vi "LSMcontroller_v58.vi"() -> ()   [LabVIEW 2015] (continued)
                    n4179 = call "2pparameters.vi"("command"="get") -> ("params out"=w943:T12)  [unwired: 1 in]
                    n4180 = Bundle By Name(cluster=w943, "Drawing Mode"=w916, "measpoints"=w932, "tt_cycles"=w934, "refreshbuffer"=w929, "refreshrate"=w928, "Vx-ref"=w935, "Vy-ref"=w937, "srate"=w926, "finite"=w939, "cont"=w938, "wavdet"=w940, "avpp"=w936, "srateAODO"=w933, "bufferAI"=w929, "bin"=w931, "Angle Img"=w923, "Vxminref"=w922, "Vxmaxref"=w921, "Vyminref"=w920, "Vymaxref"=w919, "Xpixels Img"=w918, "Ypixels Img"=w917, "Pel"=w915, "Vz-reset"=0.0, "AIoverride"=w913, "type"="Lifetime (contour)") -> (w941:T12)
                    n4181 = Reciprocal(x=w928) -> (1/x=w925:dbl)
                    n4182 = local write "refreshtime"(w925) -> ()
                    n4183 = call "2pparameters.vi"("Params in"=w941, "command"="set") -> ()  [unwired: 1 out]
                  }
                  frame "X-Y-Z-t movie" {
                  }
                  frame "linescan" {
                  }
                  frame "Timetrace" {
                    n4184 = local read "Vy-min draw"() -> (w953:dbl)
                    n4185 = local read "Vy-max draw"() -> (w952:dbl)
                    n4186 = local read "Vx-min draw"() -> (w955:dbl)
                    n4187 = local read "Vx-max draw"() -> (w954:dbl)
                    n4188 = local read "xpixels ref"() -> (w951:i32)
                    n4189 = local read "ypixels ref"() -> (w950:i32)
                    n4190 = local read "ROI Type"() -> (w949:u16)
                    n4191 = local read "srateAODOtt"() -> (w960:dbl)
                    n4192 = local read "# of frames"() -> (w965:i32)
                    n4193 = local read "refreshtime"() -> (w957:dbl)
                    n4194 = local read "Pel"() -> (w948:dbl)
                    n4195 = local read "bin"() -> (w963:dbl)
                    n4196 = local read "Override AI buffer"() -> (w946:bool)
                    n4197 = local read "finite samples"() -> (w972:bool)
                    n4198 = local read "srateAODOtt"() -> (w959:dbl)
                    n4199 = local read "srateAODOtt"() -> (w966:dbl)
                    n4200 = local read "continuous"() -> (w971:bool)
                    n4201 = local read "Angle ref"() -> (w956:dbl)
                    n4202 = local read "wavdet"() -> (w973:bool)
                    n4203 = local read "Vx-ref"() -> (w968:dbl)
                    n4204 = local read "Vy-ref"() -> (w970:dbl)
                    n4205 = local read "avpp"() -> (w969:i32)
                    n4206 = call "tt_timeandsamples.vi"("bin"=w963, "refreshtime"=w957, "srateAODOtt"=w960, "tot#ofsamples"=w965) -> ("refreshrate"=w961:dbl, "refreshbuffer"=w962:i32, "timetracecycles"=w967:i32)  [unwired: 5 in]
                    n4207 = local read "bin"() -> (w964:dbl)
                    n4208 = call "2pparameters.vi"("command"="get") -> ("params out"=w976:T12)  [unwired: 1 in]
                    n4209 = Bundle By Name(cluster=w976, "Drawing Mode"=w949, "measpoints"=w965, "tt_cycles"=w967, "refreshbuffer"=w962, "refreshrate"=w961, "Vx-ref"=w968, "Vy-ref"=w970, "srate"=w959, "finite"=w972, "cont"=w971, "wavdet"=w973, "avpp"=w969, "srateAODO"=w966, "bufferAI"=w962, "bin"=w964, "Angle Img"=w956, "Vxminref"=w955, "Vxmaxref"=w954, "Vyminref"=w953, "Vymaxref"=w952, "Xpixels Img"=w951, "Ypixels Img"=w950, "Pel"=w948, "Vz-reset"=0.0, "AIoverride"=w946, "type"="Timetrace") -> (w974:T12)
                    n4210 = Reciprocal(x=w961) -> (1/x=w958:dbl)
                    n4211 = local write "refreshtime"(w958) -> ()
                    n4212 = call "2pparameters.vi"("Params in"=w974, "command"="set") -> ()  [unwired: 1 out]
                  }
                  frame "Lifetime (point)" {
                  }
                }
              }
              frame #1 {
                w979 = FALSE ("wavdet")
                n4213 = call "2pparameters.vi"("command"="get") -> ("params out"=w983:T12)  [unwired: 1 in]
                n4214 = Bundle By Name(cluster=w983, "finite"=w979, "cont"=w979, "wavdet"=TRUE) -> (w980:T12)
                n4215 = call "2pparameters.vi"("Params in"=w980, "command"="set") -> ()  [unwired: 1 out]
              }
              frame #2 {
                n4216 = local read "DO channels"() -> (w988:u16)
                n4217 = call "2pparameters.vi"("command"="get") -> ("params out"=w990:T12)  [unwired: 1 in]
                n4218 = Unbundle By Name(w990) -> ("aDO"=w989:u32[])
                n4219 = Search 1D Array(1D array=w989, element=w988) -> (index of element=w986:i32)  [unwired: 1 in]
                n4220 = Greater?(x=w986, y=-1) -> (0:w985:bool)
                n4221 = case shown="True" w985 {
                  tunnel: w986 -> [_ w999]
                  frame False {
                  }
                  frame True {
                    n4222 = local read "Meastab"() -> (w993:enum32{"X-Y Image", "Linescan", "Timetrace"})
                    n4223 = local read "Digital padding value"() -> (w994:dbl)
                    n4224 = local read "Digital time offset (s)"() -> (w995:dbl)
                    n4225 = case shown="\"Timetrace\"" w993 {
                      tunnel: [w1000 w1001] -> w992
                      frame "X-Y Image", Default {
                        n4226 = local read "Sampling rate"() -> (w1000:dbl)
                      }
                      frame "Timetrace" {
                        n4227 = local read "srateAODOtt"() -> (w1001:dbl)
                      }
                    }
                    n4228 = local read "Digital Freq (Hz)"() -> (w997:dbl)
                    n4229 = local read "Digital phase (s)"() -> (w996:dbl)
                    n4230 = local read "Digital DC (%)"() -> (w998:dbl)
                    n4231 = call "replace DO wf param.vi"("Digital Freq (Hz)"=w997, "Digital DC (%)"=w998, "Digital phase"=w996, "Sampling frequency (Hz)"=w992, "Digital time offset (s)"=w995, "index of DO wave"=w999, "padding value"=w994) -> ()  [unwired: 4 in]
                  }
                }
              }
              frame #3 {
                n4232 = case shown="True" w1002 {
                  tunnel: w1003 -> [_ w1010]
                  frame False {
                  }
                  frame True {
                    n4233 = local read "Meastab"() -> (w1007:enum32{"X-Y Image", "Linescan", "Timetrace"})
                    n4234 = call "waveformparamsv2.vi"("command"="get") -> ("Params out"=w1026:T16)  [unwired: 4 in, 2 out]
                    n4235 = Unbundle By Name(w1026) -> ("DO parameters"=w1025:T19)
                    n4236 = property on="refwf" class="Ring (strict)"() -> ("RingText.Text"=w1032:string)  [unwired: 2 in, 2 out]
                    n4237 = case shown="\"Timetrace\"" w1007 {
                      tunnel: [w1033 w1034] -> w1006
                      frame "X-Y Image", Default {
                        n4238 = local read "Sampling rate"() -> (w1033:dbl)
                      }
                      frame "Timetrace" {
                        n4239 = local read "srateAODOtt"() -> (w1034:dbl)
                      }
                    }
                    n4240 = call "waveformsAObuffer.vi"("command"="get") -> ("AO wf out"=w1030:waveform(dbl)[])  [unwired: 1 in]
                    n4241 = call "waveformsDObuffer.vi"("command"="get") -> ("DO wf out"=w1028:digitalwaveform[])  [unwired: 1 in]
                    n4242 = call "referfencesize.vi"("Digital waveforms in"=w1028, "Analog waveforms in"=w1030, "reference waveforms to"=w1032) -> ("number of samples"=w1023:i32)  [unwired: 2 in]
                    n4243 = Index Array(array=w1025, index=w1010) -> (element=w1024:T20)
                    n4244 = call "waveformsDObuffer.vi"("command"="get") -> ("DO wf out"=w1020:digitalwaveform[])  [unwired: 1 in]
                    n4245 = call "simple digital from wf params.vi"("waveform params"=w1024, "number of samples"=w1023) -> ("digital waveform"=w1022:digitalwaveform)
                    n4246 = property on="refwf" class="Ring (strict)"() -> ("RingText.Text"=w1012:string)  [unwired: 2 in, 2 out]
                    n4247 = Replace Array Subset(array=w1020, new element=w1022, index=w1010) -> (w1011:digitalwaveform[])
                    n4248 = call "waveformsAObuffer.vi"("command"="get") -> ("AO wf out"=w1019:waveform(dbl)[])  [unwired: 1 in]
                    n4249 = local read "wavdet"() -> (w1009:bool)
                    n4250 = call "correctwaveformsizetemp.vi"("new sampling frequency (Hz)"=w1006, "start"=FALSE, "reference waveforms to"=w1012, "Analog waveforms in"=w1019, "stop"=FALSE, "Digital waveforms in"=w1011) -> ("analog wf out"=w1015:waveform(dbl)[], "Digital wf out"=w1013:digitalwaveform[], "measpoints"=w1008:i32)
                    n4251 = local write "Analog Lines Plot"(w1015) -> ()
                    n4252 = call "GetNumCamFramesv2.vi"("Digital Waveform Graph"=w1013) -> ("Numeric"=w1014:i32)  [unwired: 10 in]
                    n4253 = local write "Digital Lines Plot"(w1013) -> ()
                    n4254 = case shown="True" w1009 {
                      tunnel: w1008 -> [_ w1035]
                      frame False {
                      }
                      frame True {
                        n4255 = local write "# of frames"(w1035) -> ()
                      }
                    }
                    n4256 = call "waveformsAObuffer.vi"("AO wf in"=w1015, "command"="set") -> ()  [unwired: 1 out]
                    n4257 = call "waveformsDObuffer.vi"("DO wf in"=w1013, "command"="set") -> ()  [unwired: 1 out]
                    n4258 = local write "Total Camera Frames"(w1014) -> ()
                  }
                }
              }
              frame #4 {
                n4259 = local read "finite samples"() -> (w1036:bool)
                n4260 = local read "continuous"() -> (w1037:bool)
                n4261 = local read "wavdet"() -> (w1038:bool)
                n4262 = call "2pparameters.vi"("command"="get") -> ("params out"=w1041:T12)  [unwired: 1 in]
                n4263 = Bundle By Name(cluster=w1041, "finite"=w1036, "cont"=w1037, "wavdet"=w1038) -> (w1039:T12)
                n4264 = call "2pparameters.vi"("Params in"=w1039, "command"="set") -> ()  [unwired: 1 out]
              }
            }
          }
          event "refwf": Value Change {
            n4265 = event-data() -> ()  [unwired: 1 in, 6 out]
            n4266 = stacked-sequence {
              frame #0 {
                n4267 = local read "Measurement"() -> (w1043:T5)
                n4268 = case shown="\"X-Y-t movie\", Default" w1043 {
                  frame "X-Y-t movie", Default {
                    n4269 = local read "avpp"() -> (w1064:i32)
                    n4270 = local read "Angle ref"() -> (w1063:dbl)
                    n4271 = local read "ROI Type"() -> (w1062:u16)
                    n4272 = local read "xpixels ref"() -> (w1059:i32)
                    n4273 = local read "Vx-min ref"() -> (w1058:dbl)
                    n4274 = local read "Vx-max ref"() -> (w1057:dbl)
                    n4275 = local read "ypixels ref"() -> (w1055:i32)
                    n4276 = local read "Vy-min ref"() -> (w1056:dbl)
                    n4277 = local read "Vy-max ref"() -> (w1052:dbl)
                    n4278 = local read "Sampling rate"() -> (w1046:dbl)
                    n4279 = local read "finite samples"() -> (w1047:bool)
                    n4280 = local read "continuous"() -> (w1050:bool)
                    n4281 = local read "wavdet"() -> (w1051:bool)
                    n4282 = local read "# of frames"() -> (w1049:i32)
                    n4283 = local read "maxbufferAI"() -> (w1048:i32)
                    n4284 = local read "Override AI buffer"() -> (w1044:bool)
                    n4285 = call "2pparameters.vi"("command"="get") -> ("params out"=w1061:T12)  [unwired: 1 in]
                    n4286 = Bundle By Name(cluster=w1061, "type"="X-Y-t movie", "avpp"=w1064, "Angle Img"=w1063, "Xpixels Img"=w1059, "Vx-min Img"=w1058, "VX-max Img"=w1057, "Ypixels Img"=w1055, "Vy-min Img"=w1056, "Vy-max Img"=w1052, "srate"=w1046, "srate Img"=w1046, "finite"=w1047, "cont"=w1050, "wavdet"=w1051, "measpoints"=w1049, "maxbufferAI"=w1048, "Drawing Mode"=w1062, "Vz-reset"=0.0, "AIoverride"=w1044) -> (w1053:T12)
                    n4287 = call "2pparameters.vi"("Params in"=w1053, "command"="set") -> ()  [unwired: 1 out]
                  }
                  frame "X-Y-Z stack" {
                    n4288 = call "2pparameters.vi"("command"="get") -> ("params out"=w1068:T12)  [unwired: 1 in]
                    n4289 = Bundle By Name(cluster=w1068, "type"="X-Y-Z stack") -> (w1066:T12)
                    n4290 = call "2pparameters.vi"("Params in"=w1066, "command"="set") -> ()  [unwired: 1 out]
                  }
                  frame "Lifetime (scan)" {
                    n4291 = call "2pparameters.vi"("command"="get") -> ("params out"=w1073:T12)  [unwired: 1 in]
                    n4292 = Bundle By Name(cluster=w1073, "type"="Lifetime (scan)") -> (w1071:T12)
                    n4293 = call "2pparameters.vi"("Params in"=w1071, "command"="set") -> ()  [unwired: 1 out]
                  }
                  frame "Lifetime (contour)" {
                    n4294 = local read "Vy-min draw"() -> (w1083:dbl)
                    n4295 = local read "Vy-max draw"() -> (w1082:dbl)
                    n4296 = local read "Vx-min draw"() -> (w1085:dbl)
                    n4297 = local read "Vx-max draw"() -> (w1084:dbl)
                    n4298 = local read "xpixels ref"() -> (w1081:i32)
                    n4299 = local read "ypixels ref"() -> (w1080:i32)
                    n4300 = local read "ROI Type"() -> (w1079:u16)
                    n4301 = local read "srateAODOtt"() -> (w1090:dbl)
                    n4302 = local read "# of frames"() -> (w1095:i32)
                    n4303 = local read "refreshtime"() -> (w1087:dbl)
                    n4304 = local read "Pel"() -> (w1078:dbl)
                    n4305 = local read "bin"() -> (w1093:dbl)
                    n4306 = local read "Override AI buffer"() -> (w1076:bool)
                    n4307 = local read "finite samples"() -> (w1102:bool)
                    n4308 = local read "srateAODOtt"() -> (w1089:dbl)
                    n4309 = local read "srateAODOtt"() -> (w1096:dbl)
                    n4310 = local read "continuous"() -> (w1101:bool)
                    n4311 = local read "Angle ref"() -> (w1086:dbl)
                    n4312 = local read "wavdet"() -> (w1103:bool)
                    n4313 = local read "Vx-ref"() -> (w1098:dbl)
                    n4314 = local read "Vy-ref"() -> (w1100:dbl)
                    n4315 = local read "avpp"() -> (w1099:i32)
                    n4316 = call "tt_timeandsamples.vi"("bin"=w1093, "refreshtime"=w1087, "srateAODOtt"=w1090, "tot#ofsamples"=w1095) -> ("refreshrate"=w1091:dbl, "refreshbuffer"=w1092:i32, "timetracecycles"=w1097:i32)  [unwired: 5 in]
                    n4317 = local read "bin"() -> (w1094:dbl)
                    n4318 = call "2pparameters.vi"("command"="get") -> ("params out"=w1106:T12)  [unwired: 1 in]
                    n4319 = Bundle By Name(cluster=w1106, "Drawing Mode"=w1079, "measpoints"=w1095, "tt_cycles"=w1097, "refreshbuffer"=w1092, "refreshrate"=w1091, "Vx-ref"=w1098, "Vy-ref"=w1100, "srate"=w1089, "finite"=w1102, "cont"=w1101, "wavdet"=w1103, "avpp"=w1099, "srateAODO"=w1096, "bufferAI"=w1092, "bin"=w1094, "Angle Img"=w1086, "Vxminref"=w1085, "Vxmaxref"=w1084, "Vyminref"=w1083, "Vymaxref"=w1082, "Xpixels Img"=w1081, "Ypixels Img"=w1080, "Pel"=w1078, "Vz-reset"=0.0, "AIoverride"=w1076, "type"="Lifetime (contour)") -> (w1104:T12)
                    n4320 = Reciprocal(x=w1091) -> (1/x=w1088:dbl)
                    n4321 = local write "refreshtime"(w1088) -> ()
                    n4322 = call "2pparameters.vi"("Params in"=w1104, "command"="set") -> ()  [unwired: 1 out]
                  }
                  frame "X-Y-Z-t movie" {
                  }
                  frame "linescan" {
                  }
                  frame "Timetrace" {
                    n4323 = local read "Vy-min draw"() -> (w1116:dbl)
                    n4324 = local read "Vy-max draw"() -> (w1115:dbl)
                    n4325 = local read "Vx-min draw"() -> (w1118:dbl)
                    n4326 = local read "Vx-max draw"() -> (w1117:dbl)
                    n4327 = local read "xpixels ref"() -> (w1114:i32)
                    n4328 = local read "ypixels ref"() -> (w1113:i32)
                    n4329 = local read "ROI Type"() -> (w1112:u16)
                    n4330 = local read "srateAODOtt"() -> (w1123:dbl)
                    n4331 = local read "# of frames"() -> (w1128:i32)
                    n4332 = local read "refreshtime"() -> (w1120:dbl)
                    n4333 = local read "Pel"() -> (w1111:dbl)
                    n4334 = local read "bin"() -> (w1126:dbl)
                    n4335 = local read "Override AI buffer"() -> (w1109:bool)
                    n4336 = local read "finite samples"() -> (w1135:bool)
                    n4337 = local read "srateAODOtt"() -> (w1122:dbl)
                    n4338 = local read "srateAODOtt"() -> (w1129:dbl)
                    n4339 = local read "continuous"() -> (w1134:bool)
                    n4340 = local read "Angle ref"() -> (w1119:dbl)
                    n4341 = local read "wavdet"() -> (w1136:bool)
                    n4342 = local read "Vx-ref"() -> (w1131:dbl)
                    n4343 = local read "Vy-ref"() -> (w1133:dbl)
                    n4344 = local read "avpp"() -> (w1132:i32)
                    n4345 = call "tt_timeandsamples.vi"("bin"=w1126, "refreshtime"=w1120, "srateAODOtt"=w1123, "tot#ofsamples"=w1128) -> ("refreshrate"=w1124:dbl, "refreshbuffer"=w1125:i32, "timetracecycles"=w1130:i32)  [unwired: 5 in]
                    n4346 = local read "bin"() -> (w1127:dbl)
                    n4347 = call "2pparameters.vi"("command"="get") -> ("params out"=w1139:T12)  [unwired: 1 in]
                    n4348 = Bundle By Name(cluster=w1139, "Drawing Mode"=w1112, "measpoints"=w1128, "tt_cycles"=w1130, "refreshbuffer"=w1125, "refreshrate"=w1124, "Vx-ref"=w1131, "Vy-ref"=w1133, "srate"=w1122, "finite"=w1135, "cont"=w1134, "wavdet"=w1136, "avpp"=w1132, "srateAODO"=w1129, "bufferAI"=w1125, "bin"=w1127, "Angle Img"=w1119, "Vxminref"=w1118, "Vxmaxref"=w1117, "Vyminref"=w1116, "Vymaxref"=w1115, "Xpixels Img"=w1114, "Ypixels Img"=w1113, "Pel"=w1111, "Vz-reset"=0.0, "AIoverride"=w1109, "type"="Timetrace") -> (w1137:T12)
                    n4349 = Reciprocal(x=w1124) -> (1/x=w1121:dbl)
                    n4350 = local write "refreshtime"(w1121) -> ()
                    n4351 = call "2pparameters.vi"("Params in"=w1137, "command"="set") -> ()  [unwired: 1 out]
                  }
                  frame "Lifetime (point)" {
                  }
                }
              }
              frame #1 {
                w1142 = FALSE ("wavdet")
                n4352 = call "2pparameters.vi"("command"="get") -> ("params out"=w1146:T12)  [unwired: 1 in]
                n4353 = Bundle By Name(cluster=w1146, "finite"=w1142, "cont"=w1142, "wavdet"=TRUE) -> (w1143:T12)
                n4354 = call "2pparameters.vi"("Params in"=w1143, "command"="set") -> ()  [unwired: 1 out]
              }
              frame #2 {
                n4355 = local read "Meastab"() -> (w1151:enum32{"X-Y Image", "Linescan", "Timetrace"})
                n4356 = property on="refwf" class="Ring (strict)"() -> ("RingText.Text"=w1154:string)  [unwired: 2 in, 2 out]
                n4357 = case shown="\"Timetrace\"" w1151 {
                  tunnel: [w1164 w1165] -> w1150
                  frame "X-Y Image", Default {
                    n4358 = local read "Sampling rate"() -> (w1164:dbl)
                  }
                  frame "Timetrace" {
                    n4359 = local read "srateAODOtt"() -> (w1165:dbl)
                  }
                }
                n4360 = call "waveformsAObuffer.vi"("command"="get") -> ("AO wf out"=w1163:waveform(dbl)[])  [unwired: 1 in]
                n4361 = local read "wavdet"() -> (w1153:bool)
                n4362 = call "waveformsDObuffer.vi"("command"="get") -> ("DO wf out"=w1159:digitalwaveform[])  [unwired: 1 in]
                n4363 = call "correctwaveformsizetemp.vi"("new sampling frequency (Hz)"=w1150, "start"=FALSE, "reference waveforms to"=w1154, "Analog waveforms in"=w1163, "stop"=FALSE, "Digital waveforms in"=w1159) -> ("analog wf out"=w1157:waveform(dbl)[], "Digital wf out"=w1155:digitalwaveform[], "measpoints"=w1152:i32)
                n4364 = local write "Analog Lines Plot"(w1157) -> ()
                n4365 = call "GetNumCamFramesv2.vi"("Digital Waveform Graph"=w1155) -> ("Numeric"=w1156:i32)  [unwired: 10 in]
                n4366 = local write "Digital Lines Plot"(w1155) -> ()
                n4367 = call "waveformsDObuffer.vi"("DO wf in"=w1155, "command"="set") -> ()  [unwired: 1 out]
                n4368 = call "waveformsAObuffer.vi"("AO wf in"=w1157, "command"="set") -> ()  [unwired: 1 out]
                n4369 = local write "Total Camera Frames"(w1156) -> ()
                n4370 = case shown="True" w1153 {
                  tunnel: w1152 -> [_ w1166]
                  frame False {
                  }
                  frame True {
                    n4371 = local write "# of frames"(w1166) -> ()
                  }
                }
              }
              frame #3 {
                n4372 = local read "finite samples"() -> (w1167:bool)
                n4373 = local read "continuous"() -> (w1168:bool)
                n4374 = local read "wavdet"() -> (w1169:bool)
                n4375 = call "2pparameters.vi"("command"="get") -> ("params out"=w1172:T12)  [unwired: 1 in]
                n4376 = Bundle By Name(cluster=w1172, "finite"=w1167, "cont"=w1168, "wavdet"=w1169) -> (w1170:T12)
                n4377 = call "2pparameters.vi"("Params in"=w1170, "command"="set") -> ()  [unwired: 1 out]
              }
            }
          }
          event "Start amplitude (V)", "Cycles", "Baseline (V)", "Step size (V)", "DC (%)", "Period (ms)", "Repeats", "Pulses", "phase shift (ms)": Value Change {
            n4378 = event-data() -> ()  [unwired: 1 in, 6 out]
            n4379 = stacked-sequence {
              seq-local: [_ _ w1280 _ _] -> [_ _ _ w1302 _]
              seq-local: [_ _ w1279 _ _] -> [_ _ _ w1301 _]
              frame #0 {
                n4380 = local read "Measurement"() -> (w1174:T5)
                n4381 = case shown="\"X-Y-t movie\", Default" w1174 {
                  frame "X-Y-t movie", Default {
                    n4382 = local read "avpp"() -> (w1195:i32)
                    n4383 = local read "Angle ref"() -> (w1194:dbl)
                    n4384 = local read "ROI Type"() -> (w1193:u16)
                    n4385 = local read "xpixels ref"() -> (w1190:i32)
                    n4386 = local read "Vx-min ref"() -> (w1189:dbl)
                    n4387 = local read "Vx-max ref"() -> (w1188:dbl)
                    n4388 = local read "ypixels ref"() -> (w1186:i32)
                    n4389 = local read "Vy-min ref"() -> (w1187:dbl)
                    n4390 = local read "Vy-max ref"() -> (w1183:dbl)
                    n4391 = local read "Sampling rate"() -> (w1177:dbl)
                    n4392 = local read "finite samples"() -> (w1178:bool)
                    n4393 = local read "continuous"() -> (w1181:bool)
                    n4394 = local read "wavdet"() -> (w1182:bool)
                    n4395 = local read "# of frames"() -> (w1180:i32)
                    n4396 = local read "maxbufferAI"() -> (w1179:i32)
                    n4397 = local read "Override AI buffer"() -> (w1175:bool)
                    n4398 = call "2pparameters.vi"("command"="get") -> ("params out"=w1192:T12)  [unwired: 1 in]
                    n4399 = Bundle By Name(cluster=w1192, "type"="X-Y-t movie", "avpp"=w1195, "Angle Img"=w1194, "Xpixels Img"=w1190, "Vx-min Img"=w1189, "VX-max Img"=w1188, "Ypixels Img"=w1186, "Vy-min Img"=w1187, "Vy-max Img"=w1183, "srate"=w1177, "srate Img"=w1177, "finite"=w1178, "cont"=w1181, "wavdet"=w1182, "measpoints"=w1180, "maxbufferAI"=w1179, "Drawing Mode"=w1193, "Vz-reset"=0.0, "AIoverride"=w1175) -> (w1184:T12)
                    n4400 = call "2pparameters.vi"("Params in"=w1184, "command"="set") -> ()  [unwired: 1 out]
                  }
                  frame "X-Y-Z stack" {
                    n4401 = call "2pparameters.vi"("command"="get") -> ("params out"=w1199:T12)  [unwired: 1 in]
                    n4402 = Bundle By Name(cluster=w1199, "type"="X-Y-Z stack") -> (w1197:T12)
                    n4403 = call "2pparameters.vi"("Params in"=w1197, "command"="set") -> ()  [unwired: 1 out]
                  }
                  frame "Lifetime (scan)" {
                    n4404 = call "2pparameters.vi"("command"="get") -> ("params out"=w1204:T12)  [unwired: 1 in]
                    n4405 = Bundle By Name(cluster=w1204, "type"="Lifetime (scan)") -> (w1202:T12)
                    n4406 = call "2pparameters.vi"("Params in"=w1202, "command"="set") -> ()  [unwired: 1 out]
                  }
                  frame "Lifetime (contour)" {
                    n4407 = local read "Vy-min draw"() -> (w1214:dbl)
                    n4408 = local read "Vy-max draw"() -> (w1213:dbl)
                    n4409 = local read "Vx-min draw"() -> (w1216:dbl)
                    n4410 = local read "Vx-max draw"() -> (w1215:dbl)
                    n4411 = local read "xpixels ref"() -> (w1212:i32)
                    n4412 = local read "ypixels ref"() -> (w1211:i32)
                    n4413 = local read "ROI Type"() -> (w1210:u16)
                    n4414 = local read "srateAODOtt"() -> (w1221:dbl)
                    n4415 = local read "# of frames"() -> (w1226:i32)
                    n4416 = local read "refreshtime"() -> (w1218:dbl)
                    n4417 = local read "Pel"() -> (w1209:dbl)
                    n4418 = local read "bin"() -> (w1224:dbl)
                    n4419 = local read "Override AI buffer"() -> (w1207:bool)
                    n4420 = local read "finite samples"() -> (w1233:bool)
                    n4421 = local read "srateAODOtt"() -> (w1220:dbl)
                    n4422 = local read "srateAODOtt"() -> (w1227:dbl)
                    n4423 = local read "continuous"() -> (w1232:bool)
                    n4424 = local read "Angle ref"() -> (w1217:dbl)
                    n4425 = local read "wavdet"() -> (w1234:bool)
                    n4426 = local read "Vx-ref"() -> (w1229:dbl)
                    n4427 = local read "Vy-ref"() -> (w1231:dbl)
                    n4428 = local read "avpp"() -> (w1230:i32)
                    n4429 = call "tt_timeandsamples.vi"("bin"=w1224, "refreshtime"=w1218, "srateAODOtt"=w1221, "tot#ofsamples"=w1226) -> ("refreshrate"=w1222:dbl, "refreshbuffer"=w1223:i32, "timetracecycles"=w1228:i32)  [unwired: 5 in]
                    n4430 = local read "bin"() -> (w1225:dbl)
                    n4431 = call "2pparameters.vi"("command"="get") -> ("params out"=w1237:T12)  [unwired: 1 in]
                    n4432 = Bundle By Name(cluster=w1237, "Drawing Mode"=w1210, "measpoints"=w1226, "tt_cycles"=w1228, "refreshbuffer"=w1223, "refreshrate"=w1222, "Vx-ref"=w1229, "Vy-ref"=w1231, "srate"=w1220, "finite"=w1233, "cont"=w1232, "wavdet"=w1234, "avpp"=w1230, "srateAODO"=w1227, "bufferAI"=w1223, "bin"=w1225, "Angle Img"=w1217, "Vxminref"=w1216, "Vxmaxref"=w1215, "Vyminref"=w1214, "Vymaxref"=w1213, "Xpixels Img"=w1212, "Ypixels Img"=w1211, "Pel"=w1209, "Vz-reset"=0.0, "AIoverride"=w1207, "type"="Lifetime (contour)") -> (w1235:T12)
                    n4433 = Reciprocal(x=w1222) -> (1/x=w1219:dbl)
                    n4434 = local write "refreshtime"(w1219) -> ()
                    n4435 = call "2pparameters.vi"("Params in"=w1235, "command"="set") -> ()  [unwired: 1 out]
                  }
                  frame "X-Y-Z-t movie" {
                  }
                  frame "linescan" {
                  }
                  frame "Timetrace" {
                    n4436 = local read "Vy-min draw"() -> (w1247:dbl)
                    n4437 = local read "Vy-max draw"() -> (w1246:dbl)
                    n4438 = local read "Vx-min draw"() -> (w1249:dbl)
                    n4439 = local read "Vx-max draw"() -> (w1248:dbl)
                    n4440 = local read "xpixels ref"() -> (w1245:i32)
                    n4441 = local read "ypixels ref"() -> (w1244:i32)
                    n4442 = local read "ROI Type"() -> (w1243:u16)
                    n4443 = local read "srateAODOtt"() -> (w1254:dbl)
                    n4444 = local read "# of frames"() -> (w1259:i32)
                    n4445 = local read "refreshtime"() -> (w1251:dbl)
                    n4446 = local read "Pel"() -> (w1242:dbl)
                    n4447 = local read "bin"() -> (w1257:dbl)
                    n4448 = local read "Override AI buffer"() -> (w1240:bool)
                    n4449 = local read "finite samples"() -> (w1266:bool)
                    n4450 = local read "srateAODOtt"() -> (w1253:dbl)
                    n4451 = local read "srateAODOtt"() -> (w1260:dbl)
                    n4452 = local read "continuous"() -> (w1265:bool)
                    n4453 = local read "Angle ref"() -> (w1250:dbl)
                    n4454 = local read "wavdet"() -> (w1267:bool)
                    n4455 = local read "Vx-ref"() -> (w1262:dbl)
                    n4456 = local read "Vy-ref"() -> (w1264:dbl)
                    n4457 = local read "avpp"() -> (w1263:i32)
                    n4458 = call "tt_timeandsamples.vi"("bin"=w1257, "refreshtime"=w1251, "srateAODOtt"=w1254, "tot#ofsamples"=w1259) -> ("refreshrate"=w1255:dbl, "refreshbuffer"=w1256:i32, "timetracecycles"=w1261:i32)  [unwired: 5 in]
                    n4459 = local read "bin"() -> (w1258:dbl)
                    n4460 = call "2pparameters.vi"("command"="get") -> ("params out"=w1270:T12)  [unwired: 1 in]
                    n4461 = Bundle By Name(cluster=w1270, "Drawing Mode"=w1243, "measpoints"=w1259, "tt_cycles"=w1261, "refreshbuffer"=w1256, "refreshrate"=w1255, "Vx-ref"=w1262, "Vy-ref"=w1264, "srate"=w1253, "finite"=w1266, "cont"=w1265, "wavdet"=w1267, "avpp"=w1263, "srateAODO"=w1260, "bufferAI"=w1256, "bin"=w1258, "Angle Img"=w1250, "Vxminref"=w1249, "Vxmaxref"=w1248, "Vyminref"=w1247, "Vymaxref"=w1246, "Xpixels Img"=w1245, "Ypixels Img"=w1244, "Pel"=w1242, "Vz-reset"=0.0, "AIoverride"=w1240, "type"="Timetrace") -> (w1268:T12)
                    n4462 = Reciprocal(x=w1255) -> (1/x=w1252:dbl)
                    n4463 = local write "refreshtime"(w1252) -> ()
                    n4464 = call "2pparameters.vi"("Params in"=w1268, "command"="set") -> ()  [unwired: 1 out]
                  }
                  frame "Lifetime (point)" {
                  }
                }
              }
              frame #1 {
                w1273 = FALSE ("wavdet")
                n4465 = call "2pparameters.vi"("command"="get") -> ("params out"=w1277:T12)  [unwired: 1 in]
                n4466 = Bundle By Name(cluster=w1277, "finite"=w1273, "cont"=w1273, "wavdet"=TRUE) -> (w1274:T12)
                n4467 = call "2pparameters.vi"("Params in"=w1274, "command"="set") -> ()  [unwired: 1 out]
              }
              frame #2 {
                n4468 = local read "AO channels"() -> (w1282:u32)
                n4469 = call "2pparameters.vi"("command"="get") -> ("params out"=w1284:T12)  [unwired: 1 in]
                n4470 = Unbundle By Name(w1284) -> ("aAO"=w1283:u32[])
                n4471 = Search 1D Array(1D array=w1283, element=w1282) -> (index of element=w1280:i32)  [unwired: 1 in]
                n4472 = Greater?(x=w1280, y=-1) -> (0:w1279:bool)
                n4473 = case shown="True" w1279 {
                  tunnel: w1280 -> [_ w1298]
                  frame False {
                  }
                  frame True {
                    n4474 = local read "Meastab"() -> (w1287:enum32{"X-Y Image", "Linescan", "Timetrace"})
                    n4475 = case shown="\"Timetrace\"" w1287 {
                      tunnel: [w1299 w1300] -> w1286
                      frame "X-Y Image", Default {
                        n4476 = local read "Sampling rate"() -> (w1299:dbl)
                      }
                      frame "Timetrace" {
                        n4477 = local read "srateAODOtt"() -> (w1300:dbl)
                      }
                    }
                    n4478 = local read "Start amplitude (V)"() -> (w1295:dbl)
                    n4479 = local read "phase shift (ms)"() -> (w1290:dbl)
                    n4480 = local read "Step size (V)"() -> (w1293:dbl)
                    n4481 = local read "Baseline (V)"() -> (w1294:dbl)
                    n4482 = local read "Period (ms)"() -> (w1291:dbl)
                    n4483 = local read "padding value"() -> (w1288:dbl)
                    n4484 = local read "Repeats"() -> (w1297:dbl)
                    n4485 = local read "Cycles"() -> (w1296:dbl)
                    n4486 = local read "DC (%)"() -> (w1292:dbl)
                    n4487 = local read "Pulses"() -> (w1289:dbl)
                    n4488 = call "replace AO square wf param.vi"("Baseline (V)"=w1294, "Start amplitude (V)"=w1295, "Cycles"=w1296, "Repeats"=w1297, "index of AO wave"=w1298, "Step size (V)"=w1293, "DC (%)"=w1292, "Sampling frequency (Hz)"=w1286, "Period (ms)"=w1291, "Cycle length (s)"=w1290, "Pulses"=w1289, "padding value"=w1288) -> ()  [unwired: 4 in]
                  }
                }
              }
              frame #3 {
                n4489 = case shown="True" w1301 {
                  tunnel: w1302 -> [_ w1310]
                  frame False {
                  }
                  frame True {
                    n4490 = call "waveformparamsv2.vi"("command"="get") -> ("Params out"=w1324:T16)  [unwired: 4 in, 2 out]
                    n4491 = Unbundle By Name(w1324) -> ("AO parameters"=w1323:T17)
                    n4492 = local read "Meastab"() -> (w1305:enum32{"X-Y Image", "Linescan", "Timetrace"})
                    n4493 = case shown="\"Timetrace\"" w1305 {
                      tunnel: [w1326 w1327] -> w1314
                      frame "X-Y Image", Default {
                        n4494 = local read "Sampling rate"() -> (w1326:dbl)
                      }
                      frame "Timetrace" {
                        n4495 = local read "srateAODOtt"() -> (w1327:dbl)
                      }
                    }
                    n4496 = Index Array(array=w1323, index=w1310) -> (element=w1312:T18)
                    n4497 = call "waveformsAObuffer.vi"("command"="get") -> ("AO wf out"=w1311:waveform(dbl)[])  [unwired: 1 in]
                    n4498 = call "generateRampedSquareWave_fromAOparameters.vi"("AO params"=w1312) -> ("Waveform"=w1309:waveform(dbl))  [unwired: 1 out]
                    n4499 = property on="refwf" class="Ring (strict)"() -> ("RingText.Text"=w1313:string)  [unwired: 2 in, 2 out]
                    n4500 = Replace Array Subset(array=w1311, new element=w1309, index=w1310) -> (w1308:waveform(dbl)[])
                    n4501 = call "waveformsDObuffer.vi"("command"="get") -> ("DO wf out"=w1319:digitalwaveform[])  [unwired: 1 in]
                    n4502 = call "correctwaveformsizetemp.vi"("new sampling frequency (Hz)"=w1314, "start"=FALSE, "reference waveforms to"=w1313, "Analog waveforms in"=w1308, "stop"=FALSE, "Digital waveforms in"=w1319) -> ("analog wf out"=w1317:waveform(dbl)[], "Digital wf out"=w1315:digitalwaveform[], "measpoints"=w1306:i32)
                    n4503 = local read "wavdet"() -> (w1307:bool)
                    n4504 = local write "Analog Lines Plot"(w1317) -> ()
                    n4505 = call "GetNumCamFramesv2.vi"("Digital Waveform Graph"=w1315) -> ("Numeric"=w1316:i32)  [unwired: 10 in]
                    n4506 = local write "Digital Lines Plot"(w1315) -> ()
                    n4507 = call "waveformsAObuffer.vi"("AO wf in"=w1317, "command"="set") -> ()  [unwired: 1 out]
                    n4508 = call "waveformsDObuffer.vi"("DO wf in"=w1315, "command"="set") -> ()  [unwired: 1 out]
                    n4509 = local write "Total Camera Frames"(w1316) -> ()
                    n4510 = case shown="True" w1307 {
                      tunnel: w1306 -> [_ w1328]
                      frame False {
                      }
                      frame True {
                        n4511 = local write "# of frames"(w1328) -> ()
                      }
                    }
                  }
                }
              }
              frame #4 {
                n4512 = local read "finite samples"() -> (w1329:bool)
                n4513 = local read "continuous"() -> (w1330:bool)
                n4514 = local read "wavdet"() -> (w1331:bool)
                n4515 = call "2pparameters.vi"("command"="get") -> ("params out"=w1334:T12)  [unwired: 1 in]
                n4516 = Bundle By Name(cluster=w1334, "finite"=w1329, "cont"=w1330, "wavdet"=w1331) -> (w1332:T12)
                n4517 = call "2pparameters.vi"("Params in"=w1332, "command"="set") -> ()  [unwired: 1 out]
              }
            }
          }
          event "Amplitude (V)", "Offset (V)", "Frequency", "Tri Repeats": Value Change {
            n4518 = event-data() -> ()  [unwired: 1 in, 6 out]
            n4519 = stacked-sequence {
              seq-local: [_ _ w1442 _ _] -> [_ _ _ w1460 _]
              seq-local: [_ _ w1441 _ _] -> [_ _ _ w1459 _]
              frame #0 {
                n4520 = local read "Measurement"() -> (w1336:T5)
                n4521 = case shown="\"X-Y-t movie\", Default" w1336 {
                  frame "X-Y-t movie", Default {
                    n4522 = local read "avpp"() -> (w1357:i32)
                    n4523 = local read "Angle ref"() -> (w1356:dbl)
                    n4524 = local read "ROI Type"() -> (w1355:u16)
                    n4525 = local read "xpixels ref"() -> (w1352:i32)
                    n4526 = local read "Vx-min ref"() -> (w1351:dbl)
                    n4527 = local read "Vx-max ref"() -> (w1350:dbl)
                    n4528 = local read "ypixels ref"() -> (w1348:i32)
                    n4529 = local read "Vy-min ref"() -> (w1349:dbl)
                    n4530 = local read "Vy-max ref"() -> (w1345:dbl)
                    n4531 = local read "Sampling rate"() -> (w1339:dbl)
                    n4532 = local read "finite samples"() -> (w1340:bool)
                    n4533 = local read "continuous"() -> (w1343:bool)
                    n4534 = local read "wavdet"() -> (w1344:bool)
                    n4535 = local read "# of frames"() -> (w1342:i32)
                    n4536 = local read "maxbufferAI"() -> (w1341:i32)
                    n4537 = local read "Override AI buffer"() -> (w1337:bool)
                    n4538 = call "2pparameters.vi"("command"="get") -> ("params out"=w1354:T12)  [unwired: 1 in]
                    n4539 = Bundle By Name(cluster=w1354, "type"="X-Y-t movie", "avpp"=w1357, "Angle Img"=w1356, "Xpixels Img"=w1352, "Vx-min Img"=w1351, "VX-max Img"=w1350, "Ypixels Img"=w1348, "Vy-min Img"=w1349, "Vy-max Img"=w1345, "srate"=w1339, "srate Img"=w1339, "finite"=w1340, "cont"=w1343, "wavdet"=w1344, "measpoints"=w1342, "maxbufferAI"=w1341, "Drawing Mode"=w1355, "Vz-reset"=0.0, "AIoverride"=w1337) -> (w1346:T12)
                    n4540 = call "2pparameters.vi"("Params in"=w1346, "command"="set") -> ()  [unwired: 1 out]
                  }
                  frame "X-Y-Z stack" {
                    n4541 = call "2pparameters.vi"("command"="get") -> ("params out"=w1361:T12)  [unwired: 1 in]
                    n4542 = Bundle By Name(cluster=w1361, "type"="X-Y-Z stack") -> (w1359:T12)
                    n4543 = call "2pparameters.vi"("Params in"=w1359, "command"="set") -> ()  [unwired: 1 out]
                  }
                  frame "Lifetime (scan)" {
                    n4544 = call "2pparameters.vi"("command"="get") -> ("params out"=w1366:T12)  [unwired: 1 in]
                    n4545 = Bundle By Name(cluster=w1366, "type"="Lifetime (scan)") -> (w1364:T12)
                    n4546 = call "2pparameters.vi"("Params in"=w1364, "command"="set") -> ()  [unwired: 1 out]
                  }
                  frame "Lifetime (contour)" {
                    n4547 = local read "Vy-min draw"() -> (w1376:dbl)
                    n4548 = local read "Vy-max draw"() -> (w1375:dbl)
                    n4549 = local read "Vx-min draw"() -> (w1378:dbl)
                    n4550 = local read "Vx-max draw"() -> (w1377:dbl)
                    n4551 = local read "xpixels ref"() -> (w1374:i32)
                    n4552 = local read "ypixels ref"() -> (w1373:i32)
                    n4553 = local read "ROI Type"() -> (w1372:u16)
                    n4554 = local read "srateAODOtt"() -> (w1383:dbl)
                    n4555 = local read "# of frames"() -> (w1388:i32)
                    n4556 = local read "refreshtime"() -> (w1380:dbl)
                    n4557 = local read "Pel"() -> (w1371:dbl)
                    n4558 = local read "bin"() -> (w1386:dbl)
                    n4559 = local read "Override AI buffer"() -> (w1369:bool)
                    n4560 = local read "finite samples"() -> (w1395:bool)
                    n4561 = local read "srateAODOtt"() -> (w1382:dbl)
                    n4562 = local read "srateAODOtt"() -> (w1389:dbl)
                    n4563 = local read "continuous"() -> (w1394:bool)
                    n4564 = local read "Angle ref"() -> (w1379:dbl)
                    n4565 = local read "wavdet"() -> (w1396:bool)
                    n4566 = local read "Vx-ref"() -> (w1391:dbl)
                    n4567 = local read "Vy-ref"() -> (w1393:dbl)
                    n4568 = local read "avpp"() -> (w1392:i32)
                    n4569 = call "tt_timeandsamples.vi"("bin"=w1386, "refreshtime"=w1380, "srateAODOtt"=w1383, "tot#ofsamples"=w1388) -> ("refreshrate"=w1384:dbl, "refreshbuffer"=w1385:i32, "timetracecycles"=w1390:i32)  [unwired: 5 in]
                    n4570 = local read "bin"() -> (w1387:dbl)
                    n4571 = call "2pparameters.vi"("command"="get") -> ("params out"=w1399:T12)  [unwired: 1 in]
                    n4572 = Bundle By Name(cluster=w1399, "Drawing Mode"=w1372, "measpoints"=w1388, "tt_cycles"=w1390, "refreshbuffer"=w1385, "refreshrate"=w1384, "Vx-ref"=w1391, "Vy-ref"=w1393, "srate"=w1382, "finite"=w1395, "cont"=w1394, "wavdet"=w1396, "avpp"=w1392, "srateAODO"=w1389, "bufferAI"=w1385, "bin"=w1387, "Angle Img"=w1379, "Vxminref"=w1378, "Vxmaxref"=w1377, "Vyminref"=w1376, "Vymaxref"=w1375, "Xpixels Img"=w1374, "Ypixels Img"=w1373, "Pel"=w1371, "Vz-reset"=0.0, "AIoverride"=w1369, "type"="Lifetime (contour)") -> (w1397:T12)
                    n4573 = Reciprocal(x=w1384) -> (1/x=w1381:dbl)
                    n4574 = local write "refreshtime"(w1381) -> ()
                    n4575 = call "2pparameters.vi"("Params in"=w1397, "command"="set") -> ()  [unwired: 1 out]
                  }
                  frame "X-Y-Z-t movie" {
                  }
                  frame "linescan" {
                  }
                  frame "Timetrace" {
                    n4576 = local read "Vy-min draw"() -> (w1409:dbl)
                    n4577 = local read "Vy-max draw"() -> (w1408:dbl)
                    n4578 = local read "Vx-min draw"() -> (w1411:dbl)
                    n4579 = local read "Vx-max draw"() -> (w1410:dbl)
                    n4580 = local read "xpixels ref"() -> (w1407:i32)
                    n4581 = local read "ypixels ref"() -> (w1406:i32)
                    n4582 = local read "ROI Type"() -> (w1405:u16)
                    n4583 = local read "srateAODOtt"() -> (w1416:dbl)
                    n4584 = local read "# of frames"() -> (w1421:i32)
                    n4585 = local read "refreshtime"() -> (w1413:dbl)
                    n4586 = local read "Pel"() -> (w1404:dbl)
                    n4587 = local read "bin"() -> (w1419:dbl)
                    n4588 = local read "Override AI buffer"() -> (w1402:bool)
                    n4589 = local read "finite samples"() -> (w1428:bool)
                    n4590 = local read "srateAODOtt"() -> (w1415:dbl)
                    n4591 = local read "srateAODOtt"() -> (w1422:dbl)
                    n4592 = local read "continuous"() -> (w1427:bool)
                    n4593 = local read "Angle ref"() -> (w1412:dbl)
                    n4594 = local read "wavdet"() -> (w1429:bool)
                    n4595 = local read "Vx-ref"() -> (w1424:dbl)
                    n4596 = local read "Vy-ref"() -> (w1426:dbl)
                    n4597 = local read "avpp"() -> (w1425:i32)
                    n4598 = call "tt_timeandsamples.vi"("bin"=w1419, "refreshtime"=w1413, "srateAODOtt"=w1416, "tot#ofsamples"=w1421) -> ("refreshrate"=w1417:dbl, "refreshbuffer"=w1418:i32, "timetracecycles"=w1423:i32)  [unwired: 5 in]
                    n4599 = local read "bin"() -> (w1420:dbl)
                    n4600 = call "2pparameters.vi"("command"="get") -> ("params out"=w1432:T12)  [unwired: 1 in]
                    n4601 = Bundle By Name(cluster=w1432, "Drawing Mode"=w1405, "measpoints"=w1421, "tt_cycles"=w1423, "refreshbuffer"=w1418, "refreshrate"=w1417, "Vx-ref"=w1424, "Vy-ref"=w1426, "srate"=w1415, "finite"=w1428, "cont"=w1427, "wavdet"=w1429, "avpp"=w1425, "srateAODO"=w1422, "bufferAI"=w1418, "bin"=w1420, "Angle Img"=w1412, "Vxminref"=w1411, "Vxmaxref"=w1410, "Vyminref"=w1409, "Vymaxref"=w1408, "Xpixels Img"=w1407, "Ypixels Img"=w1406, "Pel"=w1404, "Vz-reset"=0.0, "AIoverride"=w1402, "type"="Timetrace") -> (w1430:T12)
                    n4602 = Reciprocal(x=w1417) -> (1/x=w1414:dbl)
                    n4603 = local write "refreshtime"(w1414) -> ()
                    n4604 = call "2pparameters.vi"("Params in"=w1430, "command"="set") -> ()  [unwired: 1 out]
                  }
                  frame "Lifetime (point)" {
                  }
                }
              }
              frame #1 {
                w1435 = FALSE ("wavdet")
                n4605 = call "2pparameters.vi"("command"="get") -> ("params out"=w1439:T12)  [unwired: 1 in]
                n4606 = Bundle By Name(cluster=w1439, "finite"=w1435, "cont"=w1435, "wavdet"=TRUE) -> (w1436:T12)
                n4607 = call "2pparameters.vi"("Params in"=w1436, "command"="set") -> ()  [unwired: 1 out]
              }
              frame #2 {
                n4608 = local read "AO channels"() -> (w1444:u32)
                n4609 = call "2pparameters.vi"("command"="get") -> ("params out"=w1446:T12)  [unwired: 1 in]
                n4610 = Unbundle By Name(w1446) -> ("aAO"=w1445:u32[])
                n4611 = Search 1D Array(1D array=w1445, element=w1444) -> (index of element=w1442:i32)  [unwired: 1 in]
                n4612 = Greater?(x=w1442, y=-1) -> (0:w1441:bool)
                n4613 = case shown="True" w1441 {
                  tunnel: w1442 -> [_ w1456]
                  frame False {
                  }
                  frame True {
                    n4614 = local read "Meastab"() -> (w1449:enum32{"X-Y Image", "Linescan", "Timetrace"})
                    n4615 = local read "Tri padding value"() -> (w1450:dbl)
                    n4616 = local read "Amplitude (V)"() -> (w1454:dbl)
                    n4617 = local read "Tri Phase (s)"() -> (w1451:dbl)
                    n4618 = local read "Tri Repeats"() -> (w1452:dbl)
                    n4619 = local read "Frequency"() -> (w1453:dbl)
                    n4620 = local read "Offset (V)"() -> (w1455:dbl)
                    n4621 = case shown="\"Timetrace\"" w1449 {
                      tunnel: [w1457 w1458] -> w1448
                      frame "X-Y Image", Default {
                        n4622 = local read "Sampling rate"() -> (w1457:dbl)
                      }
                      frame "Timetrace" {
                        n4623 = local read "srateAODOtt"() -> (w1458:dbl)
                      }
                    }
                    n4624 = call "replace AO tri wf param.vi"("padding value"=w1450, "index of AO wave"=w1456, "Tri phase"=w1451, "Sampling frequency (Hz)"=w1448, "Tri Repeats"=w1452, "Frequency"=w1453, "Amplitude (V)"=w1454, "Offset (V)"=w1455) -> ()
                  }
                }
              }
              frame #3 {
                n4625 = case shown="True" w1459 {
                  tunnel: w1460 -> [_ w1469]
                  frame False {
                  }
                  frame True {
                    n4626 = call "waveformparamsv2.vi"("command"="get") -> ("Params out"=w1482:T16)  [unwired: 4 in, 2 out]
                    n4627 = Unbundle By Name(w1482) -> ("AO parameters"=w1481:T17)
                    n4628 = local read "Meastab"() -> (w1464:enum32{"X-Y Image", "Linescan", "Timetrace"})
                    n4629 = case shown="\"Timetrace\"" w1464 {
                      tunnel: [w1484 w1485] -> w1463
                      frame "X-Y Image", Default {
                        n4630 = local read "Sampling rate"() -> (w1484:dbl)
                      }
                      frame "Timetrace" {
                        n4631 = local read "srateAODOtt"() -> (w1485:dbl)
                      }
                    }
                    n4632 = Index Array(array=w1481, index=w1469) -> (element=w1471:T18)
                    n4633 = call "waveformsAObuffer.vi"("command"="get") -> ("AO wf out"=w1470:waveform(dbl)[])  [unwired: 1 in]
                    n4634 = call "generateTriWave_fromAOparameters.vi"("AO params"=w1471) -> ("Waveform"=w1468:waveform(dbl))  [unwired: 1 out]
                    n4635 = property on="refwf" class="Ring (strict)"() -> ("RingText.Text"=w1472:string)  [unwired: 2 in, 2 out]
                    n4636 = Replace Array Subset(array=w1470, new element=w1468, index=w1469) -> (w1467:waveform(dbl)[])
                    n4637 = call "waveformsDObuffer.vi"("command"="get") -> ("DO wf out"=w1477:digitalwaveform[])  [unwired: 1 in]
                    n4638 = call "correctwaveformsizetemp.vi"("new sampling frequency (Hz)"=w1463, "start"=FALSE, "reference waveforms to"=w1472, "Analog waveforms in"=w1467, "stop"=FALSE, "Digital waveforms in"=w1477) -> ("analog wf out"=w1475:waveform(dbl)[], "Digital wf out"=w1473:digitalwaveform[], "measpoints"=w1465:i32)
                    n4639 = local read "wavdet"() -> (w1466:bool)
                    n4640 = local write "Analog Lines Plot"(w1475) -> ()
                    n4641 = call "GetNumCamFramesv2.vi"("Digital Waveform Graph"=w1473) -> ("Numeric"=w1474:i32)  [unwired: 10 in]
                    n4642 = local write "Digital Lines Plot"(w1473) -> ()
                    n4643 = call "waveformsAObuffer.vi"("AO wf in"=w1475, "command"="set") -> ()  [unwired: 1 out]
                    n4644 = call "waveformsDObuffer.vi"("DO wf in"=w1473, "command"="set") -> ()  [unwired: 1 out]
                    n4645 = local write "Total Camera Frames"(w1474) -> ()
                    n4646 = case shown="True" w1466 {
                      tunnel: w1465 -> [_ w1486]
                      frame False {
                      }
                      frame True {
                        n4647 = local write "# of frames"(w1486) -> ()
                      }
                    }
                  }
                }
              }
              frame #4 {
                n4648 = local read "finite samples"() -> (w1487:bool)
                n4649 = local read "continuous"() -> (w1488:bool)
                n4650 = local read "wavdet"() -> (w1489:bool)
                n4651 = call "2pparameters.vi"("command"="get") -> ("params out"=w1492:T12)  [unwired: 1 in]
                n4652 = Bundle By Name(cluster=w1492, "finite"=w1487, "cont"=w1488, "wavdet"=w1489) -> (w1490:T12)
                n4653 = call "2pparameters.vi"("Params in"=w1490, "command"="set") -> ()  [unwired: 1 out]
              }
            }
          }
          event "Load Matlab Waveform": Value Change {
            n4654 = event-data() -> ()  [unwired: 1 in, 6 out]
            n4655 = stacked-sequence {
              seq-local: [_ _ w1600 _ _] -> [_ _ _ w1615 _]
              seq-local: [_ _ w1599 _ _] -> [_ _ _ w1614 _]
              frame #0 {
                n4656 = local read "Measurement"() -> (w1494:T5)
                n4657 = case shown="\"X-Y-t movie\", Default" w1494 {
                  frame "X-Y-t movie", Default {
                    n4658 = local read "avpp"() -> (w1515:i32)
                    n4659 = local read "Angle ref"() -> (w1514:dbl)
                    n4660 = local read "ROI Type"() -> (w1513:u16)
                    n4661 = local read "xpixels ref"() -> (w1510:i32)
                    n4662 = local read "Vx-min ref"() -> (w1509:dbl)
                    n4663 = local read "Vx-max ref"() -> (w1508:dbl)
                    n4664 = local read "ypixels ref"() -> (w1506:i32)
                    n4665 = local read "Vy-min ref"() -> (w1507:dbl)
                    n4666 = local read "Vy-max ref"() -> (w1503:dbl)
                    n4667 = local read "Sampling rate"() -> (w1497:dbl)
                    n4668 = local read "finite samples"() -> (w1498:bool)
                    n4669 = local read "continuous"() -> (w1501:bool)
                    n4670 = local read "wavdet"() -> (w1502:bool)
                    n4671 = local read "# of frames"() -> (w1500:i32)
                    n4672 = local read "maxbufferAI"() -> (w1499:i32)
                    n4673 = local read "Override AI buffer"() -> (w1495:bool)
                    n4674 = call "2pparameters.vi"("command"="get") -> ("params out"=w1512:T12)  [unwired: 1 in]
                    n4675 = Bundle By Name(cluster=w1512, "type"="X-Y-t movie", "avpp"=w1515, "Angle Img"=w1514, "Xpixels Img"=w1510, "Vx-min Img"=w1509, "VX-max Img"=w1508, "Ypixels Img"=w1506, "Vy-min Img"=w1507, "Vy-max Img"=w1503, "srate"=w1497, "srate Img"=w1497, "finite"=w1498, "cont"=w1501, "wavdet"=w1502, "measpoints"=w1500, "maxbufferAI"=w1499, "Drawing Mode"=w1513, "Vz-reset"=0.0, "AIoverride"=w1495) -> (w1504:T12)
                    n4676 = call "2pparameters.vi"("Params in"=w1504, "command"="set") -> ()  [unwired: 1 out]
                  }
                  frame "X-Y-Z stack" {
                    n4677 = call "2pparameters.vi"("command"="get") -> ("params out"=w1519:T12)  [unwired: 1 in]
                    n4678 = Bundle By Name(cluster=w1519, "type"="X-Y-Z stack") -> (w1517:T12)
                    n4679 = call "2pparameters.vi"("Params in"=w1517, "command"="set") -> ()  [unwired: 1 out]
                  }
                  frame "Lifetime (scan)" {
                    n4680 = call "2pparameters.vi"("command"="get") -> ("params out"=w1524:T12)  [unwired: 1 in]
                    n4681 = Bundle By Name(cluster=w1524, "type"="Lifetime (scan)") -> (w1522:T12)
                    n4682 = call "2pparameters.vi"("Params in"=w1522, "command"="set") -> ()  [unwired: 1 out]
                  }
                  frame "Lifetime (contour)" {
                    n4683 = local read "Vy-min draw"() -> (w1534:dbl)
                    n4684 = local read "Vy-max draw"() -> (w1533:dbl)
                    n4685 = local read "Vx-min draw"() -> (w1536:dbl)
                    n4686 = local read "Vx-max draw"() -> (w1535:dbl)
                    n4687 = local read "xpixels ref"() -> (w1532:i32)
                    n4688 = local read "ypixels ref"() -> (w1531:i32)
                    n4689 = local read "ROI Type"() -> (w1530:u16)
                    n4690 = local read "srateAODOtt"() -> (w1541:dbl)
                    n4691 = local read "# of frames"() -> (w1546:i32)
                    n4692 = local read "refreshtime"() -> (w1538:dbl)
                    n4693 = local read "Pel"() -> (w1529:dbl)
                    n4694 = local read "bin"() -> (w1544:dbl)
                    n4695 = local read "Override AI buffer"() -> (w1527:bool)
                    n4696 = local read "finite samples"() -> (w1553:bool)
                    n4697 = local read "srateAODOtt"() -> (w1540:dbl)
                    n4698 = local read "srateAODOtt"() -> (w1547:dbl)
                    n4699 = local read "continuous"() -> (w1552:bool)
                    n4700 = local read "Angle ref"() -> (w1537:dbl)
                    n4701 = local read "wavdet"() -> (w1554:bool)
                    n4702 = local read "Vx-ref"() -> (w1549:dbl)
                    n4703 = local read "Vy-ref"() -> (w1551:dbl)
                    n4704 = local read "avpp"() -> (w1550:i32)
                    n4705 = call "tt_timeandsamples.vi"("bin"=w1544, "refreshtime"=w1538, "srateAODOtt"=w1541, "tot#ofsamples"=w1546) -> ("refreshrate"=w1542:dbl, "refreshbuffer"=w1543:i32, "timetracecycles"=w1548:i32)  [unwired: 5 in]
                    n4706 = local read "bin"() -> (w1545:dbl)
                    n4707 = call "2pparameters.vi"("command"="get") -> ("params out"=w1557:T12)  [unwired: 1 in]
                    n4708 = Bundle By Name(cluster=w1557, "Drawing Mode"=w1530, "measpoints"=w1546, "tt_cycles"=w1548, "refreshbuffer"=w1543, "refreshrate"=w1542, "Vx-ref"=w1549, "Vy-ref"=w1551, "srate"=w1540, "finite"=w1553, "cont"=w1552, "wavdet"=w1554, "avpp"=w1550, "srateAODO"=w1547, "bufferAI"=w1543, "bin"=w1545, "Angle Img"=w1537, "Vxminref"=w1536, "Vxmaxref"=w1535, "Vyminref"=w1534, "Vymaxref"=w1533, "Xpixels Img"=w1532, "Ypixels Img"=w1531, "Pel"=w1529, "Vz-reset"=0.0, "AIoverride"=w1527, "type"="Lifetime (contour)") -> (w1555:T12)
                    n4709 = Reciprocal(x=w1542) -> (1/x=w1539:dbl)
                    n4710 = local write "refreshtime"(w1539) -> ()
                    n4711 = call "2pparameters.vi"("Params in"=w1555, "command"="set") -> ()  [unwired: 1 out]
                  }
                  frame "X-Y-Z-t movie" {
                  }
                  frame "linescan" {
                  }
                  frame "Timetrace" {
                    n4712 = local read "Vy-min draw"() -> (w1567:dbl)
                    n4713 = local read "Vy-max draw"() -> (w1566:dbl)
                    n4714 = local read "Vx-min draw"() -> (w1569:dbl)
                    n4715 = local read "Vx-max draw"() -> (w1568:dbl)
                    n4716 = local read "xpixels ref"() -> (w1565:i32)
                    n4717 = local read "ypixels ref"() -> (w1564:i32)
                    n4718 = local read "ROI Type"() -> (w1563:u16)
                    n4719 = local read "srateAODOtt"() -> (w1574:dbl)
                    n4720 = local read "# of frames"() -> (w1579:i32)
                    n4721 = local read "refreshtime"() -> (w1571:dbl)
                    n4722 = local read "Pel"() -> (w1562:dbl)
                    n4723 = local read "bin"() -> (w1577:dbl)
                    n4724 = local read "Override AI buffer"() -> (w1560:bool)
                    n4725 = local read "finite samples"() -> (w1586:bool)
                    n4726 = local read "srateAODOtt"() -> (w1573:dbl)
                    n4727 = local read "srateAODOtt"() -> (w1580:dbl)
                    n4728 = local read "continuous"() -> (w1585:bool)
                    n4729 = local read "Angle ref"() -> (w1570:dbl)
                    n4730 = local read "wavdet"() -> (w1587:bool)
                    n4731 = local read "Vx-ref"() -> (w1582:dbl)
                    n4732 = local read "Vy-ref"() -> (w1584:dbl)
                    n4733 = local read "avpp"() -> (w1583:i32)
                    n4734 = call "tt_timeandsamples.vi"("bin"=w1577, "refreshtime"=w1571, "srateAODOtt"=w1574, "tot#ofsamples"=w1579) -> ("refreshrate"=w1575:dbl, "refreshbuffer"=w1576:i32, "timetracecycles"=w1581:i32)  [unwired: 5 in]
                    n4735 = local read "bin"() -> (w1578:dbl)
                    n4736 = call "2pparameters.vi"("command"="get") -> ("params out"=w1590:T12)  [unwired: 1 in]
                    n4737 = Bundle By Name(cluster=w1590, "Drawing Mode"=w1563, "measpoints"=w1579, "tt_cycles"=w1581, "refreshbuffer"=w1576, "refreshrate"=w1575, "Vx-ref"=w1582, "Vy-ref"=w1584, "srate"=w1573, "finite"=w1586, "cont"=w1585, "wavdet"=w1587, "avpp"=w1583, "srateAODO"=w1580, "bufferAI"=w1576, "bin"=w1578, "Angle Img"=w1570, "Vxminref"=w1569, "Vxmaxref"=w1568, "Vyminref"=w1567, "Vymaxref"=w1566, "Xpixels Img"=w1565, "Ypixels Img"=w1564, "Pel"=w1562, "Vz-reset"=0.0, "AIoverride"=w1560, "type"="Timetrace") -> (w1588:T12)
                    n4738 = Reciprocal(x=w1575) -> (1/x=w1572:dbl)
                    n4739 = local write "refreshtime"(w1572) -> ()
                    n4740 = call "2pparameters.vi"("Params in"=w1588, "command"="set") -> ()  [unwired: 1 out]
                  }
                  frame "Lifetime (point)" {
                  }
                }
              }
              frame #1 {
                w1593 = FALSE ("wavdet")
                n4741 = call "2pparameters.vi"("command"="get") -> ("params out"=w1597:T12)  [unwired: 1 in]
                n4742 = Bundle By Name(cluster=w1597, "finite"=w1593, "cont"=w1593, "wavdet"=TRUE) -> (w1594:T12)
                n4743 = call "2pparameters.vi"("Params in"=w1594, "command"="set") -> ()  [unwired: 1 out]
              }
              frame #2 {
                n4744 = local read "AO channels"() -> (w1602:u32)
                n4745 = call "2pparameters.vi"("command"="get") -> ("params out"=w1604:T12)  [unwired: 1 in]
                n4746 = Unbundle By Name(w1604) -> ("aAO"=w1603:u32[])
                n4747 = Search 1D Array(1D array=w1603, element=w1602) -> (index of element=w1600:i32)  [unwired: 1 in]
                n4748 = Greater?(x=w1600, y=-1) -> (0:w1599:bool)
                n4749 = case shown="True" w1599 {
                  tunnel: w1600 -> [_ w1611]
                  frame False {
                  }
                  frame True {
                    n4750 = local read "Meastab"() -> (w1607:enum32{"X-Y Image", "Linescan", "Timetrace"})
                    n4751 = local read "Matlab waveform path"() -> (w1609:path)
                    n4752 = local read "Matlab padding value"() -> (w1610:dbl)
                    n4753 = case shown="\"Timetrace\"" w1607 {
                      tunnel: [w1612 w1613] -> w1606
                      frame "X-Y Image", Default {
                        n4754 = local read "Sampling rate"() -> (w1612:dbl)
                      }
                      frame "Timetrace" {
                        n4755 = local read "srateAODOtt"() -> (w1613:dbl)
                      }
                    }
                    n4756 = call "matlabwfexistsdialogue.vi"("Matlab waveform path"=w1609) -> ("mtalab waveform path out"=w1608:path)
                    n4757 = call "replace AO matlab param.vi"("Sampling frequency (Hz)"=w1606, "matlab wave file"=w1608, "index of AO wave"=w1611, "padding value"=w1610) -> ()  [unwired: 7 in]
                  }
                }
              }
              frame #3 {
                n4758 = case shown="True" w1614 {
                  tunnel: w1615 -> [_ w1622]
                  frame False {
                  }
                  frame True {
                    n4759 = local read "Meastab"() -> (w1619:enum32{"X-Y Image", "Linescan", "Timetrace"})
                    n4760 = call "waveformparamsv2.vi"("command"="get") -> ("Params out"=w1625:T16)  [unwired: 4 in, 2 out]
                    n4761 = Unbundle By Name(w1625) -> ("AO parameters"=w1624:T17)
                    n4762 = case shown="\"Timetrace\"" w1619 {
                      tunnel: [w1639 w1640] -> w1618
                      frame "X-Y Image", Default {
                        n4763 = local read "Sampling rate"() -> (w1639:dbl)
                      }
                      frame "Timetrace" {
                        n4764 = local read "srateAODOtt"() -> (w1640:dbl)
                      }
                    }
